vi "STM Multi-Client - Server (RT).vi"() -> ()   [LabVIEW 2016]
uses:
  <vilib>/Platform/TimedLoop/XDataNode/XDataNode.xnode
  <vilib>/Platform/TimedLoop/XDataNode/nitl_modes.ctl
  <vilib>/Platform/TimedLoop/XDataNode/XDNodeRunTimeDep.lvlib
  <vilib>/Platform/TimedLoop/XDataNode/wakeup.ctl
  <vilib>/Platform/TimedLoop/XDataNode/timing_clust.ctl
  <vilib>/NI/STM/NI STM.lvlib
  <vilib>/NI/STM/Connection Manager/TCP/TCP Connection Method.ctl
  <vilib>/NI/STM/TCP/Write Meta Data (TCP Ref).vi
  <vilib>/NI/STM/SubVIs/MetaDataElement.ctl
  <vilib>/NI/STM/TCP/Read Message (TCP).vi
  <vilib>/NI/STM/TCP/Write Message (TCP).vi
panel:
  in  "Stop non-critical loops":bool
  out "error out":errorcluster
  out "Number of \nConnections":i32
  # "Overview: Demonstrate the use of the STM library to implement a Single Server Multi Client application design. \nRequirements: LabVIEW Full Development System, STM Library version 3.x or later\nInstructions: \n1. Run the STM Multi-Client - Server (RT) VI\n2. Set the Target IP Address in the STM Multi-Client - Client VI to match the IP address of the server\n3. Run the STM Multi-Client - Client VI\n4. Change the Channel to choose between four different waveform"
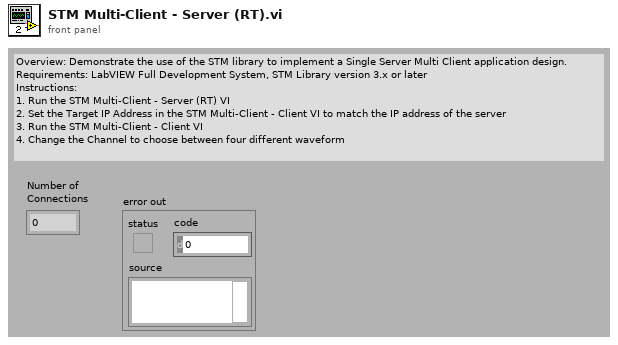
[diagram p1: front panel]
types:
  T1 = typedef "NI STM.lvlib/MetaDataElement.ctl" = string
  T2 = typedef "NI STM.lvlib/TCP Connection Method.ctl" = enum16{"Initialize", "Add Connection", "Set Properties", "Get Connection(s)", "Remove Connection", "Remove All Connections", "Get Connection Count"}
  T3 = typedef "RT FIFOs (STM Multi-Client).ctl" = cluster{"Data FIFO":T4, "Stop FIFO":T5}
  T4 = typedef "NI_Real-Time Libraries.lvlib/RTFIFORefnum DBLA.ctl" = cluster{"index":u32, "id":u32, "type":dbl[], "size":u32}
  T5 = typedef "NI_Real-Time Libraries.lvlib/RTFIFORefnum BOOL.ctl" = cluster{"index":u32, "id":u32, "type":bool, "size":u32}
  T6 = typedef "XDNodeRunTimeDep.lvlib/timing_clust.ctl" = cluster{"Expected End [f-1]":u64, "Actual End [f-1]":u64, "Finished Late? [f-1]":bool, "Expected End [i-1]":u64, "Actual End [i-1]":u64, "Finished Late? [i-1]":bool, "Expected Start [i]":u64, "Actual Start [i]":u64, "Expected Start [f]":u64, "Actual Start [f]":u64, "Source Name":string, "Structure Name":string, "Period":i64, "Deadline":i64, "Offset":i64, "Start":i64, "Priority":i32, "Timeout":i32, "Mode":T7, "Wakeup Reason":T8, "Error":errorcluster, "Source Type":string, "Secondary Source Type":string, "Global End Time":u64, "Global Start Time":u64, "Frame Duration":u64, "Iteration Duration":u64, "Assigned CPU":i32, "I/O Scan Engine Mode":u32}
  T7 = typedef "XDNodeRunTimeDep.lvlib/nitl_modes.ctl" = enum32{"No Change", "Process missed periods, maintain original phase", "Discard missed periods, maintain original phase", "Process missed periods, ignore original phase", "Discard missed periods, ignore original phase"}
  T8 = typedef "XDNodeRunTimeDep.lvlib/wakeup.ctl" = enum32{"Normal", "Aborted", "Asynchronous wakeup", "Timing source error", "Timed loop error", "Timeout"}
  T9 = typedef "NI STM.lvlib/TCP Connection Info.ctl" = cluster{"connection ID":refnum<k5>, "meta data":T1[]}
  T10 = typedef "NI STM.lvlib/TCP Connection Properties.ctl" = cluster{"Name":string, "Address":string, "Custom":string}
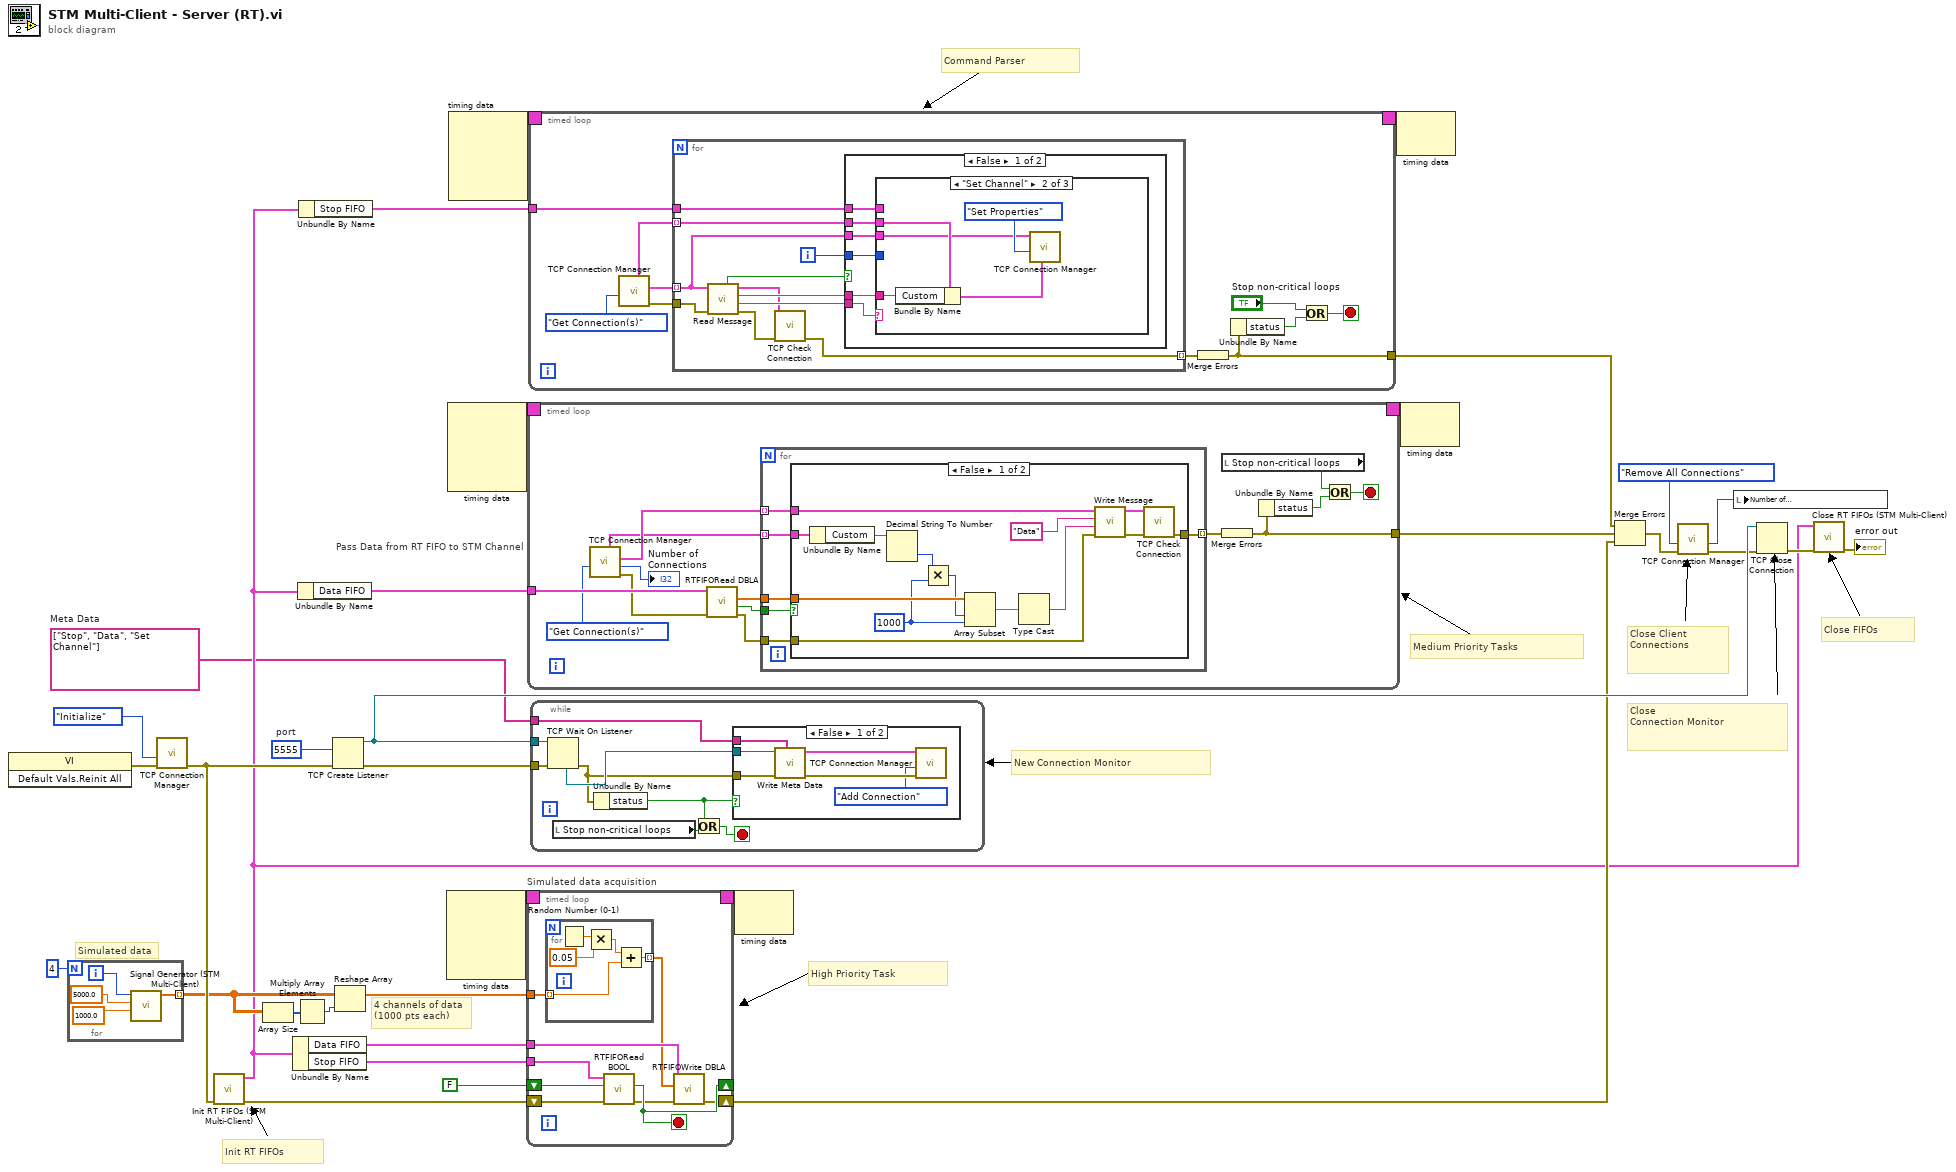
[diagram p0: block diagram]
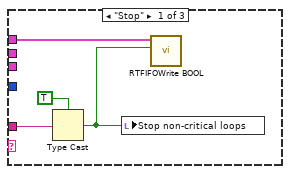
[diagram p3: hidden frame]
diagram:
  w1 = T1[] ["Stop", "Data", "Set Channel"]  # Meta Data
  w31 = u16 5555  # port
  # "4 channels of data\n(1000 pts each)"
  # "Command Parser"
  # "Medium Priority Tasks"
  # "Close \nConnection Monitor"
  # "Init RT FIFOs"
  # "Simulated data"
  # "New Connection Monitor"
  # "Close Client\nConnections"
  # "Close FIFOs"
  # "High Priority Task"
  n1 = invoke class="VI" method="Default Vals.Reinit All"() -> (error out=w7:errorcluster)  [unwired: 3 in, 2 out]
  n2 = for {
    N: 4 -> [_]
    tunnel: [w37] -> w17 mode=indexing
    i -> [w38]
    n3 = call "Signal Generator (STM Multi-Client).vi"("#Samples"=1000.0, "frequency"=5000.0, "Signal Type"=w38) -> ("Data"=w37:dbl[])  [unwired: 7 in, 1 out]
  }
  n4 = call <vilib>:"TCP Connection Manager.vi"("error in"=w7, "method"=TCP_Connection_Method."Initialize") -> ("error out"=w29:errorcluster)  [unwired: 4 in, 5 out]
  n5 = call "Init RT FIFOs (STM Multi-Client).vi"("error in (no error)"=w29) -> ("error out"=w10:errorcluster, "FIFOs out"=w8:T3)  [unwired: 9 in]
  n6 = Array Size(array=w17) -> (size(s)=w16:i32[])
  n7 = Unbundle By Name(w8) -> ("Data FIFO"=w12:T4, "Stop FIFO"=w13:T5)
  n8 = Multiply Array Elements(1:w16) -> (0:w15:i32)
  n9 = Unbundle By Name(w8) -> ("Data FIFO"=w27:T4)
  n10 = Unbundle By Name(w8) -> ("Stop FIFO"=w26:T5)
  n11 = TCP Create Listener(8:w29, 10:w31) -> (0:w32:errorcluster, 3:w30:refnum<k5>)  [unwired: 3 in, 1 out]
  n12 = Reshape Array(w17, w15) -> (w14:dbl[])
  n13 = node-c288() -> (w20:T6)  [unwired: 4 in]
  n14 = node-c288() -> (w22:T6)  [unwired: 4 in]
  n15 = node-c288() -> (w24:T6)  [unwired: 4 in]
  n16 = timed-loop "Simulated data acquisition" {
    tunnel: w14 -> [w40]
    tunnel: w13 -> [w47]
    tunnel: w12 -> [w43]
    shift-right: [w45] -> _
    shift-left: FALSE -> [w46]
    timing: w20 -> [_]
    timing-out: [_] -> w19
    shift-right: [w41] -> w9
    shift-left: w10 -> [w44]
    stop <- w45 stop-if-true
    n17 = for {
      tunnel: w40 -> [w49] mode=indexing
      tunnel: [w48] -> w39 mode=indexing
      n18 = Random Number (0-1)() -> (number: 0 to 1=w52:dbl)
      n19 = Multiply(x=w52, y=0.05) -> (x*y=w50:dbl)
      n20 = Add(x=w50, y=w49) -> (x+y=w48:dbl)
    }
    n21 = call <vilib>:"RTFIFORead BOOL.vi"("error in (no error)"=w44, "element"=w46, "rt fifo"=w47) -> ("error out"=w42:errorcluster, "element out"=w45:bool)  [unwired: 5 in, 2 out]
    n22 = call <vilib>:"RTFIFOWrite DBLA.vi"("error in (no error)"=w42, "element"=w39, "rt fifo"=w43) -> ("error out"=w41:errorcluster)  [unwired: 6 in, 2 out]
  }
  n23 = timed-loop "Pass Data from RT FIFO to STM Channel" {
    tunnel: [w62] -> w34
    tunnel: w27 -> [w60]
    timing: w22 -> [_]
    timing-out: [_] -> w21
    stop <- w68 stop-if-true
    n24 = call <vilib>:"TCP Connection Manager.vi"("method"=TCP_Connection_Method."Get Connection(s)") -> ("error out"=w56:errorcluster, "number of connections"=→"Number of \nConnections":i32, "all connections"=w65:T9[], "all properties"=w61:T10[])  [unwired: 5 in, 2 out]
    n25 = call <vilib>:"RTFIFORead DBLA.vi"("error in (no error)"=w56, "rt fifo"=w60) -> ("error out"=w55:errorcluster, "empty"=w58:bool, "element out"=w59:dbl[])  [unwired: 6 in, 1 out]
    n26 = for {
      tunnel: [w73] -> w64 mode=indexing
      tunnel: w65 -> [w74] mode=indexing
      tunnel: w61 -> [w72] mode=indexing
      tunnel: w59 -> [w71]
      tunnel: w58 -> [w70]
      tunnel: w55 -> [w69]
      n27 = case shown="False" w70 {
        tunnel: w74 -> [w77 _]
        tunnel: [w86 _] -> w73
        tunnel: w71 -> [w84 _]
        tunnel: w72 -> [w83 _]
        tunnel: w69 -> [w75 _]
        frame False {
          w82 = 1000 ("length")
          n28 = Unbundle By Name(w83) -> ("Custom"=w81:string)
          n29 = Decimal String To Number(string=w81) -> (number=w78:i32)  [unwired: 2 in, 1 out]
          n30 = Multiply(x=w78, y=w82) -> (x*y=w80:i32)
          n31 = Array Subset(array=w84, index=w80, length=w82) -> (w79:dbl[])
          n32 = Type Cast(x=w79) -> (*(type *) &x=w85:string)  [unwired: 1 in]
          n33 = call-poly <vilib>:"Write Message.vi"("error in"=w75, "data"=w85, "name"="Data" ("Name"), "connection info in"=w77) -> ("error out"=w87:errorcluster, "connection info out"=w76:T9)  [unwired: 6 in]
          n34 = call <vilib>:"TCP Check Connection.vi"("error in"=w87, "connection in"=w76) -> ("error out"=w86:errorcluster)  [unwired: 7 in, 2 out]
        }
        frame True {
        }
      }
    }
    n35 = local read "Stop non-critical loops"() -> (w66:bool)
    n36 = Merge Errors(w64) -> (w62:errorcluster)
    n37 = Unbundle By Name(w62) -> ("status"=w67:bool)
    n38 = Or(x=w66, y=w67) -> (x .or. y?=w68:bool)
  }
  n39 = timed-loop {
    tunnel: [w97] -> w33
    tunnel: w26 -> [w95]
    timing: w24 -> [_]
    timing-out: [_] -> w23
    stop <- w100 stop-if-true
    n40 = call <vilib>:"TCP Connection Manager.vi"("method"=TCP_Connection_Method."Get Connection(s)") -> ("error out"=w91:errorcluster, "all connections"=w96:T9[], "all properties"=w94:T10[])  [unwired: 5 in, 3 out]
    n41 = for {
      tunnel: [w107] -> w98 mode=indexing
      tunnel: w96 -> [w102] mode=indexing
      tunnel: w95 -> [w106]
      tunnel: w94 -> [w104] mode=indexing
      tunnel: w91 -> [w101]
      i -> [w105]
      n42 = call-poly <vilib>:"Read Message.vi"("error in"=w101, "connection info in"=w102) -> ("error out"=w108:errorcluster, "name"=w111:T1, "data string"=w110:string, "connection info out"=w103:T9, "timed out?"=w109:bool)  [unwired: 4 in, 1 out]
      n43 = call <vilib>:"TCP Check Connection.vi"("error in"=w108, "connection in"=w103) -> ("error out"=w107:errorcluster)  [unwired: 7 in, 2 out]
      n44 = case shown="False" w109 {
        tunnel: w111 -> [w112 _]
        tunnel: w110 -> [w117 _]
        tunnel: w106 -> [w116 _]
        tunnel: w102 -> [w115 _]
        tunnel: w105 -> [w114 _]
        tunnel: w104 -> [w113 _]
        frame False {
          n45 = case shown="\"Set Channel\"" w112 {
            tunnel: w117 -> [w121 w122 _]
            tunnel: w116 -> [w118 _ _]
            tunnel: w115 -> [_ w123 _]
            tunnel: w114 -> [_ _ _]
            tunnel: w113 -> [_ w126 _]
            frame "Stop" {
              n46 = Type Cast(type=TRUE, x=w121) -> (*(type *) &x=w119:bool)
              n47 = local write "Stop non-critical loops"(w119) -> ()
              n48 = call <vilib>:"RTFIFOWrite BOOL.vi"("element"=w119, "rt fifo"=w118) -> ()  [unwired: 7 in, 3 out]
            }
            frame "Set Channel" {
              n49 = Bundle By Name(cluster=w126, "Custom"=w122) -> (w125:T10)
              n50 = call <vilib>:"TCP Connection Manager.vi"("properties in"=w125, "method"=TCP_Connection_Method."Set Properties", "connection in"=w123) -> ()  [unwired: 3 in, 6 out]
            }
            frame Default {
            }
          }
        }
        frame True {
        }
      }
    }
    n51 = Merge Errors(w98) -> (w97:errorcluster)
    n52 = Unbundle By Name(w97) -> ("status"=w99:bool)
    n53 = Or(x="Stop non-critical loops", y=w99) -> (x .or. y?=w100:bool)
  }
  n54 = while "Listen loop.  Append new connections to a synchronized queue." {
    tunnel: w30 -> [w135]
    tunnel: w32 -> [w136]
    tunnel: w1 -> [w132]
    stop <- w130 stop-if-true
    n55 = TCP Wait On Listener(8:w136, 11:w135) -> (0:w131:errorcluster, 4:w134:refnum<k5>)  [unwired: 2 in, 3 out]
    n56 = local read "Stop non-critical loops"() -> (w129:bool)
    n57 = Unbundle By Name(w131) -> ("status"=w133:bool)
    n58 = Or(x=w133, y=w129) -> (x .or. y?=w130:bool)
    n59 = case shown="False" w133 {
      tunnel: w134 -> [w142 _]
      tunnel: w132 -> [w137 _]
      tunnel: w131 -> [w140 _]
      frame False {
        n60 = call-poly <vilib>:"Write Meta Data.vi"("meta data"=w137, "error in"=w140, "connection ID"=w142) -> ("error out"=w141:errorcluster, "connection info out"=w138:T9)  [unwired: 7 in]
        n61 = call <vilib>:"TCP Connection Manager.vi"("error in"=w141, "method"=TCP_Connection_Method."Add Connection", "connection in"=w138) -> ()  [unwired: 3 in, 6 out]
      }
      frame True {
      }
    }
  }
  n62 = node-c288(w19) -> ()  [unwired: 1 out]
  n63 = node-c288(w23) -> ()  [unwired: 1 out]
  n64 = node-c288(w21) -> ()  [unwired: 1 out]
  n65 = Merge Errors(w33, w34, w9) -> (w6:errorcluster)
  n66 = call <vilib>:"TCP Connection Manager.vi"("error in"=w6, "method"=TCP_Connection_Method."Remove All Connections") -> ("error out"=w5:errorcluster, "number of connections"=w4:i32)  [unwired: 4 in, 4 out]
  n67 = local write "Number of \nConnections"(w4) -> ()
  n68 = TCP Close Connection(connection ID=w30, error in (no error)=w5) -> (error out=w28:errorcluster)  [unwired: 1 in, 1 out]
  n69 = call "Close RT FIFOs (STM Multi-Client).vi"("error in (no error)"=w28, "FIFOs In"=w8) -> ("error out"=→"error out":errorcluster)  [unwired: 9 in]
